vi "http connection handler.vi"(8 "http responder":refnum<class "http responder.lvclass">, 9 "remote address":string, 10 "server properties":T1={"max url size"=8000, "max header"=8000, "timeout ms"=5000, "max data size"=104857600}, 11 "connection":refnum<k5>) -> ()   [LabVIEW 2016, in "Basic HTTP server.lvclass"]
uses:
  Basic HTTP server.lvclass
  http server properties.ctl
  HTTP responder/http responder.lvclass
  http parse state.ctl
  http request.ctl
  http method.ctl
  http header data.ctl
  http response.ctl
  http response packet type.ctl
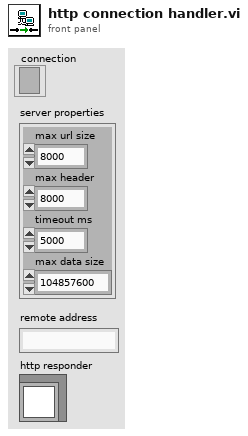
[diagram p1: front panel]
types:
  T1 = typedef "Basic HTTP server.lvclass/http server properties.ctl" = cluster{"max url size":i32, "max header":i32, "timeout ms":i32, "max data size":i32}
  T2 = typedef "Basic HTTP server.lvclass/http response.ctl" = cluster{"packet type":T3, "reason code":u16, "status string":string, "headers":T4, "cookies":string[], "data":string}
  T3 = typedef "Basic HTTP server.lvclass/http response packet type.ctl" = enum16{"full response", "header only", "data only", "last data"}
  T4 = typedef "Basic HTTP server.lvclass/http header data.ctl" = cluster{"fields":string[], "values":string[]}
  T5 = typedef "Basic HTTP server.lvclass/http request.ctl" = cluster{"remote address":string, "method":T6, "target":string, "version":string, "headers":T4, "data":string, "has data?":bool}
  T6 = typedef "Basic HTTP server.lvclass/http method.ctl" = enum16{"GET", "POST", "PUT", "DELETE", "HEAD", "OPTIONS", "upgrade"}
  T7 = typedef "Basic HTTP server.lvclass/http parse state.ctl" = enum16{"function", "headers", "data"}
  T8 = enum16{"Standard", "Buffered", "CRLF", "Immediate"}
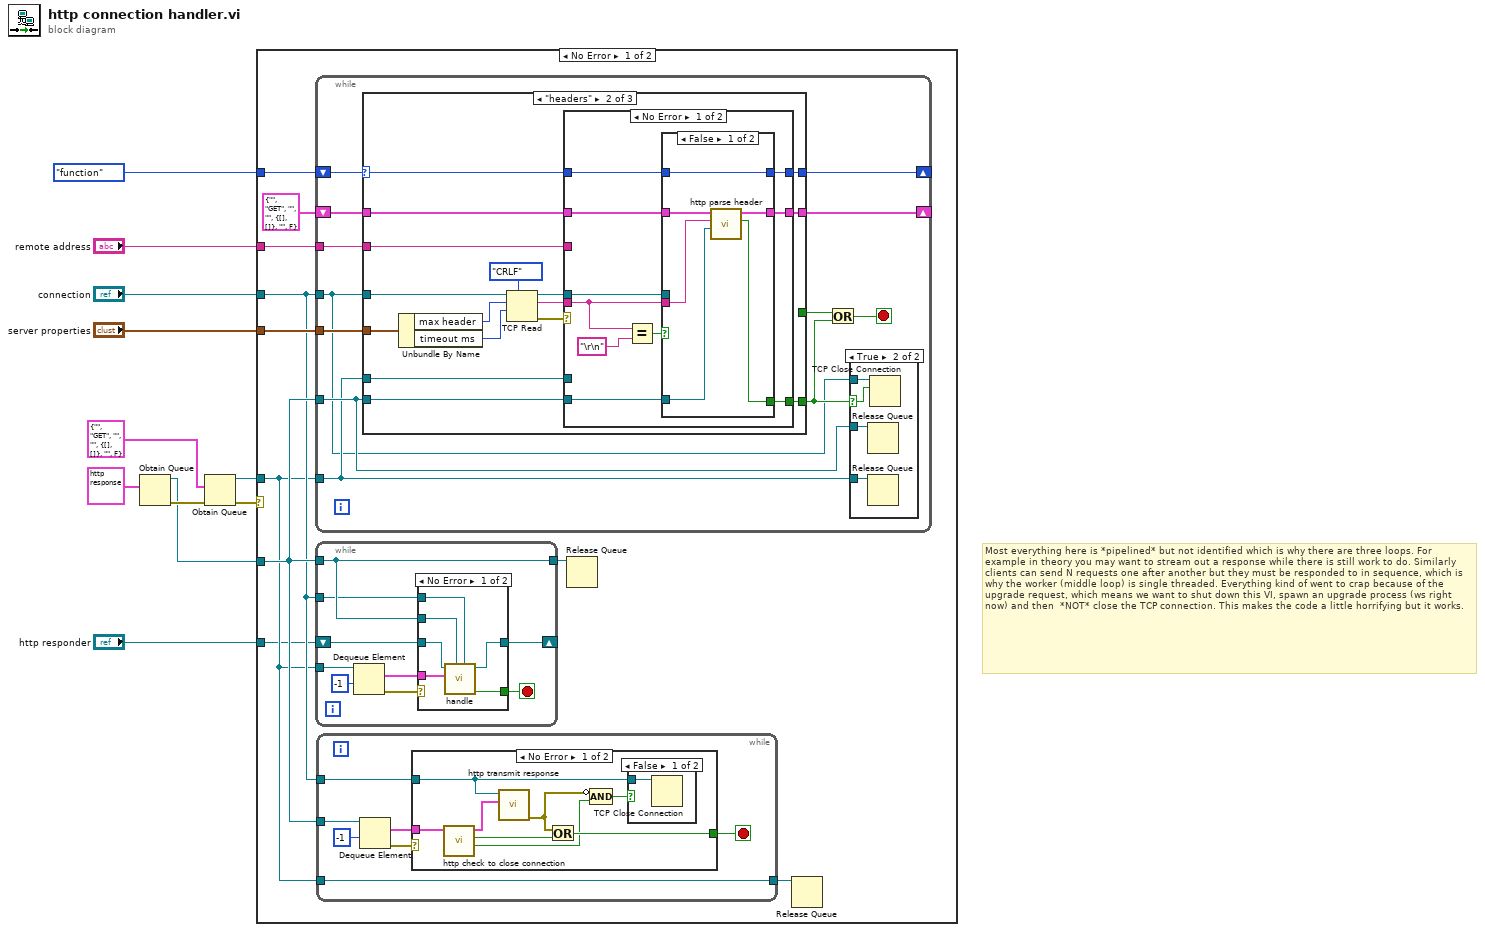
[diagram p0: block diagram]
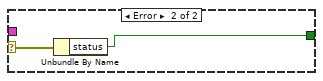
[diagram p3: hidden frame]
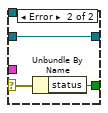
[diagram p4: hidden frame]
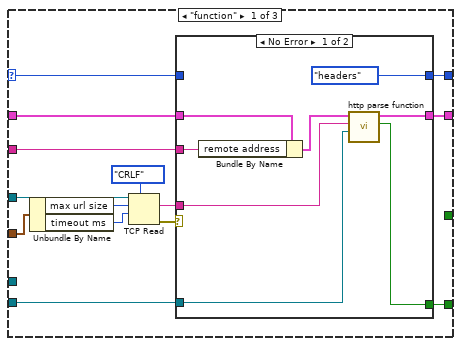
[diagram p6: hidden frame]
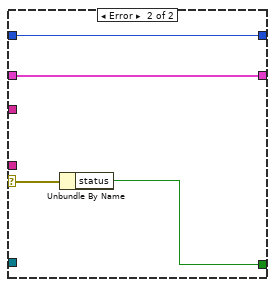
[diagram p7: hidden frame]
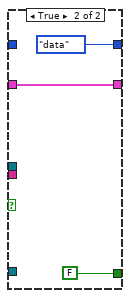
[diagram p8: hidden frame]
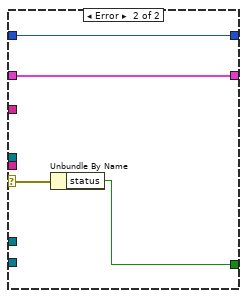
[diagram p9: hidden frame]
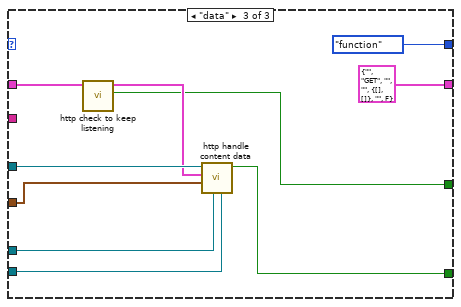
[diagram p10: hidden frame]
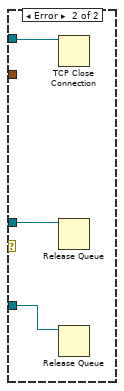
[diagram p11: hidden frame]
diagram:
  # "Most everything here is *pipelined* but not identified which is why there are three loops. For example in theory you may want to stream out a response while there is still work to do. Similarly clients can send N requests one after another but they must be responded to in sequence, which is why the worker (middle loop) is single threaded. Everything kind of went to crap because of the upgrade request, which means we want to shut down this VI, spawn an upgrade process (ws right now) and then  *NOT* close the TCP connection. This makes the code a little horrifying but it works."
  n1 = Obtain Queue(element data type=T2 {"packet type"=enum."full response", "reason code"=0, "status string"="", "headers"={"fields"=[], "values"=[]}, "cookies"=[], "data"=""} ("application request")) -> (queue out=w2:refnum<queue>, error out=w7:errorcluster)  [unwired: 4 in, 1 out]
  n2 = Obtain Queue(element data type=T5 {"remote address"="", "method"=enum."GET", "target"="", "version"="", "headers"={"fields"=[], "values"=[]}, "data"="", "has data?"=FALSE} ("application request"), error in (no error)=w7) -> (queue out=w3:refnum<queue>, error out=w9:errorcluster)  [unwired: 3 in, 1 out]
  n3 = case shown="No Error" w9 {
    tunnel: http_parse_state."function" -> [w21 _]
    tunnel: "connection" -> [w15 w151]
    tunnel: "remote address" -> [w20 _]
    tunnel: w3 -> [w14 w150]
    tunnel: "server properties" -> [w18 _]
    tunnel: w2 -> [w16 w149]
    tunnel: "http responder" -> [w12 _]
    frame No Error {
      n4 = while {
        tunnel: w15 -> [w58]
        shift-right: [w68] -> _
        shift-left: T5 {"remote address"="", "method"=enum."GET", "target"="", "version"="", "headers"={"fields"=[], "values"=[]}, "data"="", "has data?"=FALSE} ("application request") -> [w69]
        tunnel: w14 -> [w60]
        shift-right: [w67] -> _
        shift-left: w21 -> [w64]
        tunnel: w20 -> [w66]
        tunnel: w18 -> [w65]
        tunnel: w16 -> [w61]
        stop <- w63 stop-if-true
        n5 = case shown="\"headers\"" w64 {
          selector: w64 -> [w77 w103 _]
          tunnel: w69 -> [w87 w115 w141]
          tunnel: [w86 w114 T5 {"remote address"="", "method"=enum."GET", "target"="", "version"="", "headers"={"fields"=[], "values"=[]}, "data"="", "has data?"=FALSE} ("application request")] -> w68
          tunnel: w58 -> [w83 w111 w145]
          tunnel: [w81 w109 http_parse_state."function"] -> w67
          tunnel: [w80 w108 w146] -> w62
          tunnel: w66 -> [w79 w106 _]
          tunnel: w60 -> [_ w105 w143]
          tunnel: w65 -> [w76 w102 w144]
          tunnel: w61 -> [w78 w104 w142]
          tunnel: [_ _ w139] -> w59
          frame "function" {
            n6 = Unbundle By Name(w76) -> ("max url size"=w75:i32, "timeout ms"=w74:i32)
            n7 = TCP Read(connection ID=w83, bytes to read=w75, 7:T8."CRLF" ("mode (standard)"), 9:w74) -> (data out=w82:string, error out=w84:errorcluster)  [unwired: 1 in, 1 out]
            n8 = case shown="No Error" w84 {
              selector: w84 -> [_ w98]
              tunnel: w87 -> [w92 w99]
              tunnel: [w93 w99] -> w86
              tunnel: [w91 w96] -> w80
              tunnel: w82 -> [w95 _]
              tunnel: w77 -> [_ w97]
              tunnel: [http_parse_state."headers" w97] -> w81
              tunnel: w79 -> [w90 _]
              tunnel: w78 -> [w89 _]
              frame No Error {
                n9 = Bundle By Name(cluster=w92, "remote address"=w90) -> (w88:T5)
                n10 = call "http parse function.vi"("transmit queue"=w89, "data in"=w95, "application request in"=w88) -> ("abort"=w91:bool, "application request out"=w93:T5)  [unwired: 7 in]
              }
              frame Error {
                n11 = Unbundle By Name(w98) -> ("status"=w96:bool)
              }
            }
          }
          frame "headers" {
            n12 = Unbundle By Name(w102) -> ("max header"=w101:i32, "timeout ms"=w100:i32)
            n13 = TCP Read(connection ID=w111, bytes to read=w101, 7:T8."CRLF" ("mode (standard)"), 9:w100) -> (connection ID out=w107:refnum<k5>, data out=w110:string, error out=w112:errorcluster)  [unwired: 1 in]
            n14 = case shown="No Error" w112 {
              selector: w112 -> [_ w137]
              tunnel: w115 -> [w121 w138]
              tunnel: [w122 w138] -> w114
              tunnel: [w120 w135] -> w108
              tunnel: w105 -> [_ _]
              tunnel: w110 -> [w124 _]
              tunnel: w103 -> [w125 w136]
              tunnel: [w123 w136] -> w109
              tunnel: w107 -> [w119 _]
              tunnel: w106 -> [_ _]
              tunnel: w104 -> [w118 _]
              frame No Error {
                n15 = Equal?(x=w124, y="\r\n" ("x")) -> (x = y?=w116:bool)
                n16 = case shown="False" w116 {
                  tunnel: w124 -> [w130 _]
                  tunnel: w121 -> [w129 w133]
                  tunnel: [w128 w133] -> w122
                  tunnel: w125 -> [w131 _]
                  tunnel: [w131 http_parse_state."data"] -> w123
                  tunnel: [w127 FALSE ("abort")] -> w120
                  tunnel: w119 -> [_ _]
                  tunnel: w118 -> [w126 _]
                  frame False {
                    n17 = call "http parse header.vi"("transmit queue"=w126, "data in"=w130, "application request"=w129) -> ("abort"=w127:bool, "application request out"=w128:T5)  [unwired: 7 in]
                  }
                  frame True {
                  }
                }
              }
              frame Error {
                n18 = Unbundle By Name(w137) -> ("status"=w135:bool)
              }
            }
          }
          frame "data" {
            n19 = call "http check to keep listening.vi"("application request in"=w141) -> ("stop listening"=w139:bool, "application request out"=w140:T5)  [unwired: 9 in]
            n20 = call "http handle content data.vi"("transmit queue"=w142, "exec queue"=w143, "server properties"=w144, "application request"=w140, "TCP Network Connection in"=w145) -> ("abort"=w146:bool)  [unwired: 6 in]
          }
        }
        n21 = Or(x=w59, y=w62) -> (x .or. y?=w63:bool)
        n22 = case shown="True" w62 {
          selector: w62 -> [_ w71]
          tunnel: w61 -> [_ w73]
          tunnel: w60 -> [_ w72]
          tunnel: w58 -> [_ w70]
          frame False {
          }
          frame True {
            n23 = Release Queue(queue=w73) -> ()  [unwired: 2 in, 3 out]
            n24 = Release Queue(queue=w72) -> ()  [unwired: 2 in, 3 out]
            n25 = TCP Close Connection(connection ID=w70, abort (F)=w71) -> ()  [unwired: 1 in, 2 out]
          }
        }
      }
      n26 = while {
        tunnel: w16 -> [w43]
        tunnel: [w43] -> w17
        tunnel: w14 -> [w48]
        tunnel: w15 -> [w42]
        shift-right: [w40] -> _
        shift-left: w12 -> [w41]
        stop <- w45 stop-if-true
        n27 = Dequeue Element(queue=w48, timeout in ms (-1)=-1) -> (element=w44:T5, error out=w46:errorcluster)  [unwired: 1 in, 2 out]
        n28 = case shown="No Error" w46 {
          selector: w46 -> [_ w57]
          tunnel: [w50 w56] -> w45
          tunnel: w44 -> [w51 _]
          tunnel: w43 -> [w54 _]
          tunnel: w42 -> [w49 _]
          tunnel: w41 -> [w53 w55]
          tunnel: [w52 w55] -> w40
          frame No Error {
            n29 = call "handle.vi"("TCP connection"=w49, "response queue"=w54, "application request in"=w51, "http responder in"=w53) -> ("stop processing"=w50:bool, "http responder out"=w52:refnum<class "http responder.lvclass">)  [unwired: 6 in]
          }
          frame Error {
            n30 = Unbundle By Name(w57) -> ("status"=w56:bool)
          }
        }
      }
      n31 = while {
        tunnel: w15 -> [w23]
        tunnel: w16 -> [w28]
        tunnel: [w22] -> w13
        tunnel: w14 -> [w22]
        stop <- w25 stop-if-true
        n32 = Dequeue Element(queue=w28, timeout in ms (-1)=-1) -> (element=w24:T2, error out=w26:errorcluster)  [unwired: 1 in, 2 out]
        n33 = case shown="No Error" w26 {
          selector: w26 -> [_ w39]
          tunnel: [w32 w38] -> w25
          tunnel: w24 -> [w36 _]
          tunnel: w23 -> [w33 _]
          frame No Error {
            n34 = call "http check to close connection.vi"("application request"=w36) -> ("leave connection open?"=w30:bool, "stop process?"=w34:bool, "application request out"=w35:T2)  [unwired: 8 in]
            n35 = call "http transmit response.vi"("application request"=w35, "tcp connection"=w33) -> ("error out"=w29:errorcluster)  [unwired: 9 in]
            n36 = Or(x=w29, y=w34) -> (x .or. y?=w32:bool)
            n37 = Compound Arithmetic op=AND(invert w29, w30) -> (w31:bool)
            n38 = case shown="False" w31 {
              tunnel: w33 -> [w37 _]
              frame False {
                n39 = TCP Close Connection(connection ID=w37) -> ()  [unwired: 2 in, 2 out]
              }
              frame True {
              }
            }
          }
          frame Error {
            n40 = Unbundle By Name(w39) -> ("status"=w38:bool)
          }
        }
      }
      n41 = Release Queue(queue=w17) -> ()  [unwired: 2 in, 3 out]
      n42 = Release Queue(queue=w13) -> ()  [unwired: 2 in, 3 out]
    }
    frame Error {
      n43 = TCP Close Connection(connection ID=w151) -> ()  [unwired: 2 in, 2 out]
      n44 = Release Queue(queue=w150) -> ()  [unwired: 2 in, 3 out]
      n45 = Release Queue(queue=w149) -> ()  [unwired: 2 in, 3 out]
    }
  }
